vi "Read timeouts.vi"(8 "error in (no error)":errorcluster, 11 "SP in":refnum<class "Save messages PGserver.lvclass">) -> (0 "error out":errorcluster, 2 "SP timeouts":T1={"reconn_timeout"=3000, "read_timeout"=1000, "N attempt max"=3, "t_reset_TTL"=120000, "period"=100} {"read_timeout" min=1 max=5 step=1; "t_reset_TTL" min=10 max=100000 step=1; "period" min=10 max=100000 step=1; "N attempt max" min=10 max=240000 step=1; "reconn_timeout" min=10 max=240000 step=1}, 3 "SP out":refnum<class "Save messages PGserver.lvclass">)   [LabVIEW 2019, in "Save messages PGserver.lvclass"]
uses:
  Save messages PGserver.lvclass
  ctl/Save_prog_timeouts.ctl
  Save messages PGserver.lvclass/Save messages PGserver.ctl
  PostgreSQL.lvlib
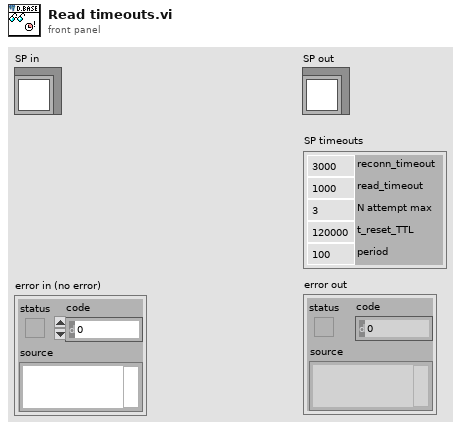
[diagram p1: front panel]
types:
  T1 = typedef "PostgreSQL.lvlib/Save_prog_timeouts.ctl" = cluster{"reconn_timeout":i32, "read_timeout":i32, "N attempt max":i32, "t_reset_TTL":i32, "period":i32}
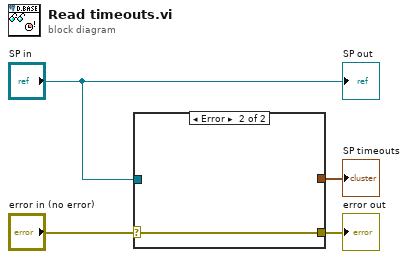
[diagram p0: block diagram]
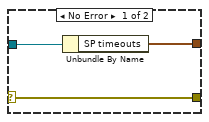
[diagram p2: hidden frame]
diagram:
  n1 = case shown="Error" "error in (no error)" {
    selector: "error in (no error)" -> [w5 w8]
    tunnel: [w5 w8] -> w3
    tunnel: "SP in" -> [w7 _]
    tunnel: [w6 _] -> w2
    frame No Error {
      n2 = Unbundle By Name(w7) -> ("SP timeouts"=w6:T1)
    }
    frame Error {
    }
  }
  "error out" <- w3
  "SP timeouts" <- w2
  "SP out" <- "SP in"
